vi "Analog_All_VI.vi"   [LabVIEW 2020]
uses:
  Available Analog Commands.ctl
  Global Analog.vi
panel:
  # "PI GCS2 LabVIEW analog driver content (disable)"
  # "This VI contains all low VIs valid for a disabled PI GCS2 analog driver. See diagram for a survey of all PI GCS2 low level VIs. Menu / Browse / Show VI Hierarchy will show the file paths of the VIs. Global Variables are shown as Control as well as Indicator."
types:
  T1 = typedef "Available Analog Commands.ctl" = enum16{"INITIALIZE", "VOL?", "VOL ", "CLOSE", "MOV", "POS?", "VCO", "VCO?", "WAIT_WF", "TMN?", "TMX?", "VEL", "VEL?", "SAI?", "MVR", "ERR?", "#24", "STP", "*IDN?", "#5", "STE", "DRR?", "W_Wave", "HLP?", "W/R_Wave"}
  T2 = cluster{"Conversion factor":dbl[], "Velocity":dbl[], "Velocity control mode":bool, "AO.Resolution":dbl, "Lower voltage limit (V)":dbl, "Upper voltage limit (V)":dbl, "AO_WF_T (s)":dbl, "AI Sample Rate":dbl, "AI Samples/Channel":i32, "Hyperbit":bool, "Offset (V)":dbl[], "Hyperbit StayOnPos":bool, "Gain (V)":dbl[], "Bit rate (Hz)":dbl, "PWM rate (Hz)":dbl, "HyperBit Password":string, "AO.MaxRate":dbl, "Conversion offset":dbl[]}[]
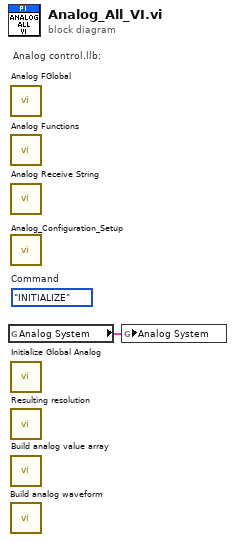
[diagram p0: block diagram]
diagram:
  (unwired) Available_Analog_Commands."INITIALIZE"  # Command
  # "Analog control.llb:"
  n1 = global read "Global Analog.vi" "Analog System"() -> (w1:T2)
  n2 = call "Analog FGlobal.vi"() -> ()  [unwired: 3 in, 17 out]
  n3 = call "Analog Functions.vi"() -> ()  [unwired: 7 in, 13 out]
  n4 = call "Analog Receive String.vi"() -> ()  [unwired: 5 in, 15 out]
  n5 = call "Analog_Configuration_Setup.vi"() -> ()  [unwired: 15 in, 5 out]
  n6 = call "Initialize Global Analog.vi"() -> ()  [unwired: 2 in, 18 out]
  n7 = call "Resulting resolution.vi"() -> ()  [unwired: 5 in, 15 out]
  n8 = call "Build analog value array.vi"() -> ()  [unwired: 11 in, 9 out]
  n9 = call "Build analog waveform.vi"() -> ()  [unwired: 5 in, 15 out]
  n10 = global write "Global Analog.vi" "Analog System"(w1) -> ()
